vi "get ancestor distance.vi"(8 "error in (no error)":errorcluster, 9 "Degree in (0)":i32, 10 "node 2":T1, 11 "node 1":T1) -> (0 "error out":errorcluster, 1 "Degree out":i32, 2 "node 2 out":T1, 3 "node 1 out":T1)   [LabVIEW 2015, in "E2E Tag Exchange editor node.lvclass"]
uses:
  E2E Tag Exchange editor node.lvclass
  <vilib>/NI/Configuration Framework/Node/NodeRef.ctl
  <vilib>/NI/Configuration Framework/Node/NISE_CEF_Node.lvclass
  <vilib>/NI/Configuration Framework/Node/NISE_CEF_Node.lvclass/NISE_CEF_Node.ctl
  <vilib>/NI/Configuration Framework/Node/ReadParent.vi
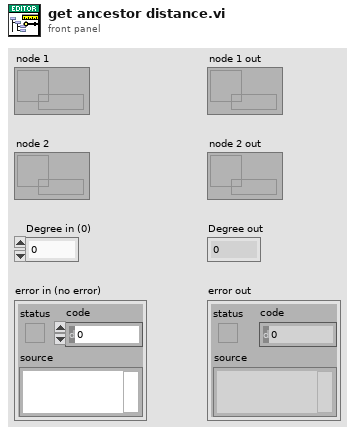
[diagram p1: front panel]
types:
  T1 = typedef "NISE_CEF_Node.lvclass/NodeRef.ctl" = refnum<data-value>
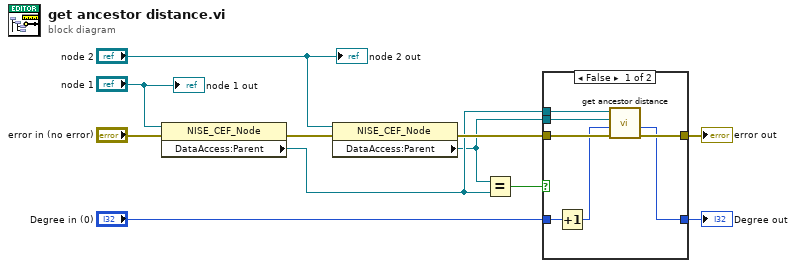
[diagram p0: block diagram]
diagram:
  n1 = property class="NISE_CEF_Node"(reference="node 1", error in="error in (no error)") -> (error out=w9:errorcluster, "DataAccess:Parent"=w2:T1)  [unwired: 1 out]
  n2 = property class="NISE_CEF_Node"(reference="node 2", error in=w9) -> (error out=w7:errorcluster, "DataAccess:Parent"=w1:T1)  [unwired: 1 out]
  n3 = Equal?(x=w1, y=w2) -> (x = y?=w6:bool)
  n4 = case shown="False" w6 {
    tunnel: w7 -> [w18 w20]
    tunnel: [w17 w20] -> w5
    tunnel: "Degree in (0)" -> [w16 w19]
    tunnel: [w14 w19] -> w3
    tunnel: w2 -> [w13 _]
    tunnel: w1 -> [w12 _]
    frame False {
      n5 = Increment(x=w16) -> (x+1=w15:i32)
      n6 = call "get ancestor distance.vi"("error in (no error)"=w18, "Degree in (0)"=w15, "node 2"=w12, "node 1"=w13) -> ("error out"=w17:errorcluster, "Degree out"=w14:i32)  [unwired: 4 in, 2 out]
    }
    frame True {
    }
  }
  "error out" <- w5
  "Degree out" <- w3
  "node 1 out" <- "node 1"
  "node 2 out" <- "node 2"
